vi "closeEMCY.vi"(8 "error in (no error)":errorcluster, 10 "emergency object in":refnum<k20>, 11 "MotorController in":refnum<class "MotorController.lvclass">) -> (0 "error out":errorcluster, 3 "MotorController out":refnum<class "MotorController.lvclass">)   [LabVIEW 2017, in "MotorController.lvclass"]
uses:
  MotorController.lvclass
  <vilib>/CANopenLib/CANOPEN.llb/CANopen Emergency Close.vi
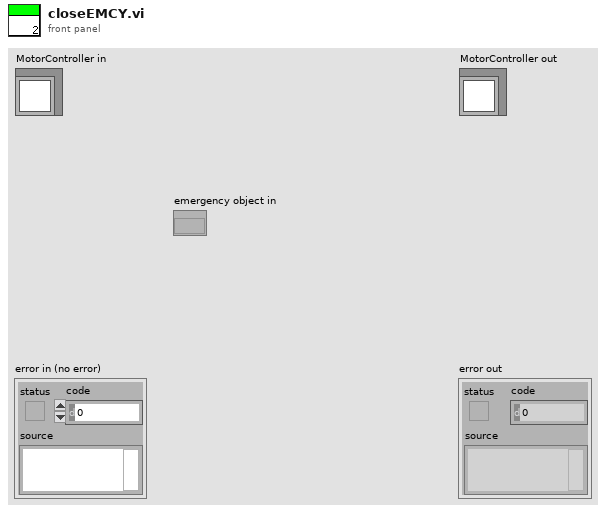
[diagram p1: front panel]
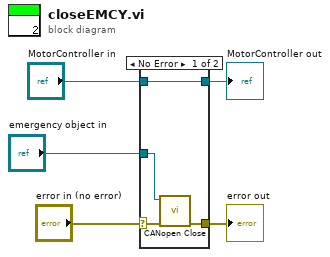
[diagram p0: block diagram]
diagram:
  n1 = case shown="No Error" "error in (no error)" {
    selector: "error in (no error)" -> [w8 w11]
    tunnel: [w7 w11] -> w4
    tunnel: [w6 w10] -> w2
    tunnel: "MotorController in" -> [w6 w10]
    tunnel: "emergency object in" -> [w9 _]
    frame No Error {
      n2 = call-poly <vilib>:"CANopen Close.vi"("error in (no error)"=w8, "emergency object in"=w9) -> ("error out"=w7:errorcluster)  [unwired: 9 in]
    }
    frame Error {
    }
  }
  "error out" <- w4
  "MotorController out" <- w2
